vi "Send Visualise FFT.vi"(6 "Frequency Metedata":T1, 7 "Message Priority (Normal)":T5=enum."Normal", 8 "error in (no error)":errorcluster, 9 "Signal Density Plot":T2, 10 "FFT Data":T4, 11 "Message Enqueuer":refnum<class "Message Enqueuer.lvclass">) -> (0 "error out":errorcluster, 3 "Message Enqueuer out":refnum<class "Message Enqueuer.lvclass">)   [LabVIEW 2025, in "UI Root.lvlib" / "Visualise FFT Msg.lvclass"]
doc: "This VI sends the message to an actor."
uses:
  Visualise FFT Msg.lvclass
  <vilib>/ActorFramework/Message Enqueuer/Message Enqueuer.lvclass
  <vilib>/ActorFramework/Message Enqueuer/Message Priority.ctl
  UI Root/FFT Plot Data.ctl
  UI Root/Signal Density Plot Data.ctl
  <vilib>/Utility/miscctls.llb/LVOffsetAndMultiplierTypeDef.ctl
  UI Root/Frequency Metadata.ctl
  C:/Program Files/National Instruments/LabVIEW 2025/vi.lib/ActorFramework/Message/Message.lvclass
  Visualise FFT Msg.lvclass/Visualise FFT Msg.ctl
  <vilib>/ActorFramework/Message Enqueuer/Message Enqueuer.lvclass/Message Enqueuer.ctl
  <vilib>/ActorFramework/Message Priority Queue/Priority Enqueue.vi
  UI Root/UI Root.lvclass
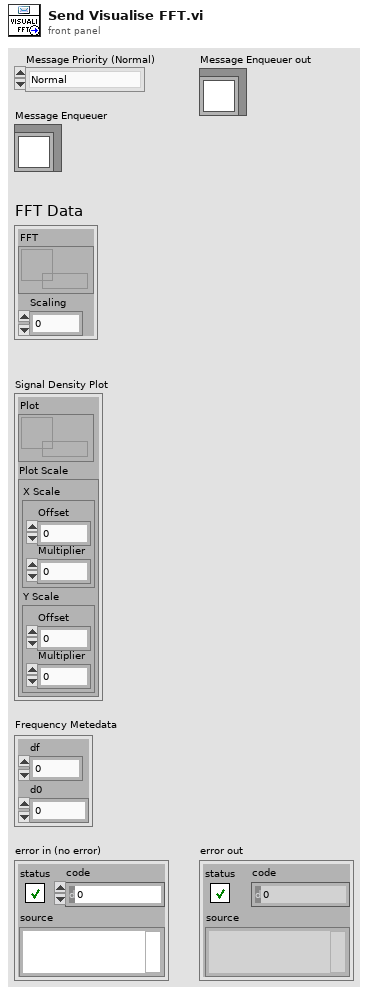
[diagram p1: front panel]
types:
  T1 = typedef "UI Root.lvlib/UI Root.lvclass/Frequency Metadata.ctl" = cluster{"df":dbl, "d0":dbl}
  T2 = typedef "UI Root.lvlib/UI Root.lvclass/Signal Density Plot Data.ctl" = cluster{"Plot":refnum<data-value>, "Plot Scale":cluster{"X Scale":T3, "Y Scale":T3}}
  T3 = typedef "LVOffsetAndMultiplierTypeDef.ctl" = cluster{"Offset":dbl, "Multiplier":dbl}
  T4 = typedef "UI Root.lvlib/UI Root.lvclass/FFT Plot Data.ctl" = cluster{"FFT":refnum<data-value>, "Scaling":dbl}
  T5 = typedef "Actor Framework.lvlib/Message Enqueuer.lvclass/Message Priority.ctl" = enum16{"Low", "Normal", "High"}
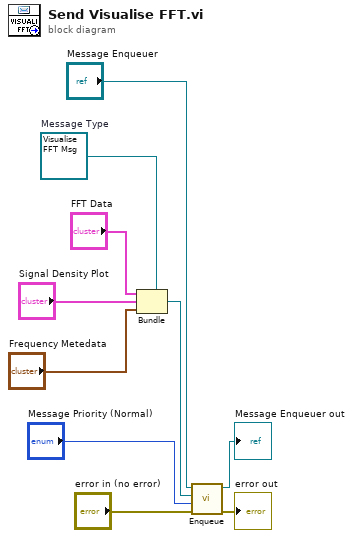
[diagram p0: block diagram]
diagram:
  w4 = refnum<class "Visualise FFT Msg.lvclass"> refnum  # Message Type
  n1 = Bundle(cluster=w4, "FFT Data", "Signal Density Plot", "Frequency Metedata") -> (w5:refnum<class "Visualise FFT Msg.lvclass">)
  n2 = call <vilib>:"Enqueue.vi"("error in (no error)"="error in (no error)", "Message Priority (Normal)"="Message Priority (Normal)", "Message"=w5, "Message Enqueuer in"="Message Enqueuer") -> ("error out"=→"error out":errorcluster, "Message Enqueuer out"=→"Message Enqueuer out":refnum<class "Message Enqueuer.lvclass">)  [unwired: 6 in]
